vi "RichToFlatstreamai_samplingConfig.vi"(5 "OutputClusterType":T1, 11 "InputCluster":T2) -> (3 "OutputCluster":T1)   [LabVIEW 2023, in "Generated_server.lvlib"]
uses:
  Generated_server.lvlib
  streamai_samplingConfig.ctl
  streamai_samplingConfig_Flat.ctl
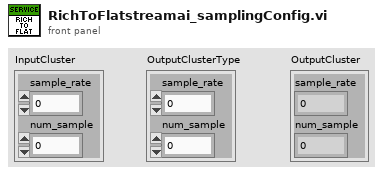
[diagram p1: front panel]
types:
  T1 = typedef "Generated_server.lvlib/streamai_samplingConfig_Flat.ctl" = cluster{"sample_rate":dbl, "num_sample":i32}
  T2 = typedef "Generated_server.lvlib/streamai_samplingConfig.ctl" = cluster{"sample_rate":dbl, "num_sample":i32}
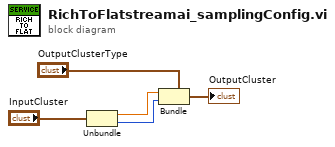
[diagram p0: block diagram]
diagram:
  n1 = Unbundle "Unbundle"("InputCluster") -> ("sample_rate"=w2:dbl, "num_sample"=w1:i32)
  n2 = Bundle "Bundle"(cluster="OutputClusterType", "sample_rate"=w2, "num_sample"=w1) -> (→"OutputCluster":T1)
